vi "TSPopup.Show Popup.vi"(6 "Font Size":u32, 8 "error in (no error)":errorcluster, 9 "Call Data (ignore if empty)":variant, 11 "Popup Parameters":T1) -> (0 "error out":errorcluster)   [LabVIEW 2013]
doc: "Invokes the Type Sensitive Popup using the provided Parameters. This <B>MUST</B> be used in the 'Mouse Down<B>?</B>' event, which is the filtering event. This makes the popup visible before allowing the mouse click to be handled.\n\n<B>Popup Parameters</B> - Parameters for showing the Type Sensitive Popup.\n<B>Call data</B> - This input will be returned with the 'Popup Event' for use in handling the Popup results.\n<B>Font Size</B> - If wired, this sets the font size of popups.\n\nType Sensitive Popup \nCopyright © 2007, J. David Saunders\nAll rights reserved."
uses:
  TSPopup.Popup Call Parameters.ctl
  TSPopup.Data Type.ctl
  Private/TSPopup.Popup Operation.ctl
panel:
  # "Type Sensitive Popup \nCopyright © 2007, J. David Saunders\nAll rights reserved."
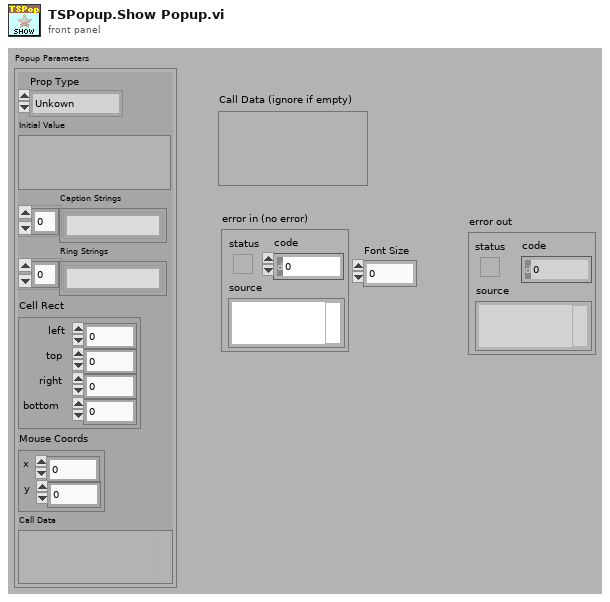
[diagram p1: front panel]
types:
  T1 = typedef "TSPopup.Popup Call Parameters.ctl" = cluster{"Prop Type":T2, "Initial Value":variant, "Caption Strings":string[], "Ring Strings":string[], "Cell Rect":cluster{"left":i16, "top":i16, "right":i16, "bottom":i16}, "Mouse Coords":cluster{"x":i16, "y":i16}, "Call Data":variant}
  T2 = typedef "TSPopup.Data Type.ctl" = enum16{"Unkown", "NO POPUP", "String", "Integer", "Float", "Color", "Boolean", "Ring", "Captioned String", "Captioned Integer", "Button Color", "2 Int Cluster", "4 Int Cluster"}
  T3 = typedef "TSPopup.Popup Operation.ctl" = enum16{"Show", "Initialize", "Close", "Popup Done", "Register a Location's Type", "Retrieve Location's Type"}
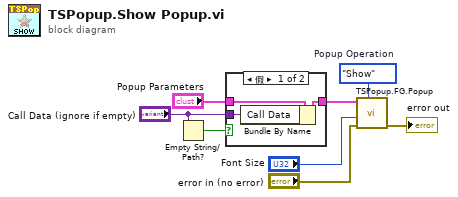
[diagram p0: block diagram]
diagram:
  w8 = TSPopup.Popup_Operation."Show"  # Popup Operation
  n1 = Empty String/Path?(string/path="Call Data (ignore if empty)") -> (empty?=w5:bool)
  n2 = case shown="假" w5 {
    tunnel: "Popup Parameters" -> [w10 w12]
    tunnel: "Call Data (ignore if empty)" -> [w11 _]
    tunnel: [w9 w12] -> w2
    frame False {
      n3 = Bundle By Name(cluster=w10, "Call Data"=w11) -> (w9:T1)
    }
    frame True {
    }
  }
  n4 = call "TSPopup.FG.Popup.vi"("Popup Operation"=w8, "error in (no error)"="error in (no error)", "Font Size"="Font Size", "Popup Parameters"=w2) -> ("error out"=→"error out":errorcluster)  [unwired: 4 in, 3 out]
